vi "connectionPoints.vi"(2 "r":T1 {"height" format="%.2f"; "width" format="%.2f"; "y" format="%.2f"; "x" format="%.2f"}, 5 "error in (no error)":errorcluster) -> (15 "path":T2[](array[typedef]) {"y" format="%.2f"; "x" format="%.2f"}, 19 "error out":errorcluster)   [LabVIEW 2020, in "BentStyle.lvclass"]
doc: "/**\n Gets the four connecting points at which a bent line\n connects to a rectangle.\n */\n private static Point2D[] connectionPoints(Rectangle2D r)"
uses:
  <resource>/Framework/Providers/Open_GDS/UML/BentStyle_class/BentStyle.lvclass
  <resource>/Framework/Providers/Open_GDS/UML/General/Point/Point Point2D.ctl
  <resource>/Framework/Providers/Open_GDS/UML/General/Rectangle/Rectangle Rectangle2D.ctl
panel:
  # "private static Point2D[] connectionPoints(Rectangle2D r)"
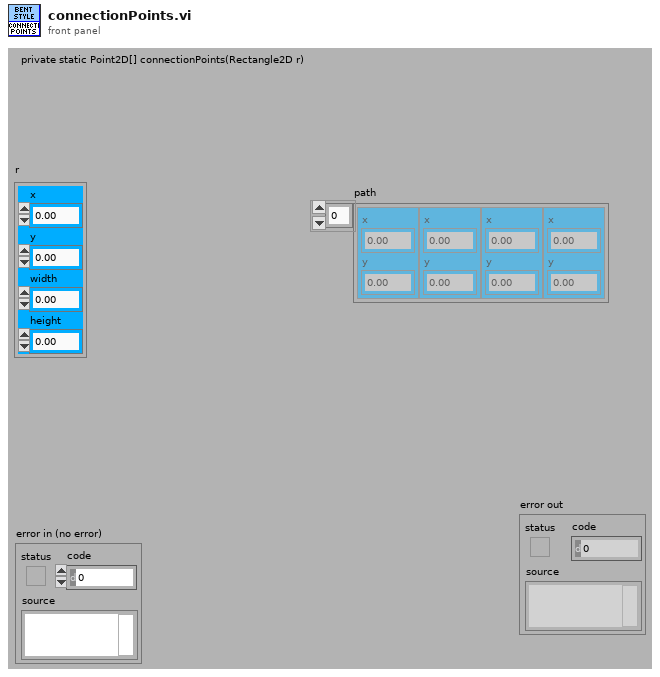
[diagram p1: front panel]
types:
  T1 = typedef "Rectangle Rectangle2D.ctl" = cluster{"x":dbl, "y":dbl, "width":dbl, "height":dbl}
  T2 = typedef "Point Point2D.ctl" = cluster{"x":dbl, "y":dbl}
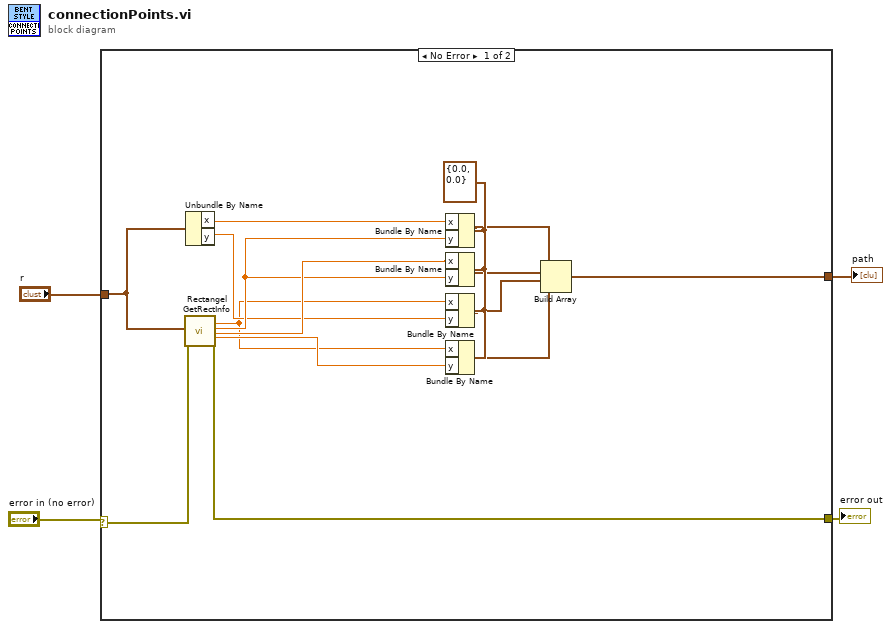
[diagram p0: block diagram]
diagram:
  n1 = case shown="No Error" "error in (no error)" {
    selector: "error in (no error)" -> [w18 w20]
    tunnel: [w17 w20] -> w4
    tunnel: "r" -> [w11 _]
    tunnel: [w12 _] -> w1
    frame No Error {
      w19 = T2 {"x"=0.0, "y"=0.0} ("point2D")
      n2 = call <resource>:"Rectangel GetRectInfo.vi"("bounds"=w11, "error in (no error)"=w18) -> ("centerX"=w5:dbl, "centerY"=w8:dbl, "maxX"=w9:dbl, "maxY"=w7:dbl, "error out"=w17:errorcluster)  [unwired: 13 out]
      n3 = Unbundle By Name(w11) -> ("x"=w10:dbl, "y"=w6:dbl)
      n4 = Bundle By Name(cluster=w19, "x"=w10, "y"=w8) -> (w16:T2)
      n5 = Bundle By Name(cluster=w19, "x"=w9, "y"=w8) -> (w15:T2)
      n6 = Bundle By Name(cluster=w19, "x"=w5, "y"=w6) -> (w14:T2)
      n7 = Bundle By Name(cluster=w19, "x"=w5, "y"=w7) -> (w13:T2)
      n8 = Build Array(w16, w15, w14, w13) -> (w12:T2[])
    }
    frame Error {
    }
  }
  "error out" <- w4
  "path" <- w1
